vi "RandomArray.vi"(11 "Numeric":i32) -> (3 "Array":dbl[](array[numeric]))   [LabVIEW 2014]
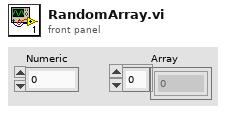
[diagram p1: front panel]
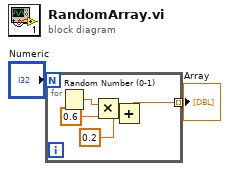
[diagram p0: block diagram]
diagram:
  n1 = for {
    N: "Numeric" -> [_]
    tunnel: [w7] -> w2 mode=indexing
    n2 = Random Number (0-1)() -> (number: 0 to 1=w6:dbl)
    n3 = Multiply(x=w6, y=0.6) -> (x*y=w5:dbl)
    n4 = Add(x=w5, y=0.2 ("x*y")) -> (x+y=w7:dbl)
  }
  "Array" <- w2
